vi "Dashboard Main KB.vi"() -> ()   [LabVIEW 2014]
uses:
  Typedefs/StackerStates.ctl
  Typedefs/Arm States.ctl
  Typedefs/ClawStates.ctl
  <vilib>/Rock Robotics/Network Tables/SD Read Boolean.vi
  <vilib>/Rock Robotics/Network Tables/SD Read Number.vi
  <vilib>/Rock Robotics/Network Tables/SD Read String Array.vi
panel:
  out "Claw On":bool
  out "Intake On":bool
  out "Right Throttle":dbl
  out "Comp Bot":bool
  out "Intake Sensor Enabled":bool
  out "Number of Totes":u8
  out "Compressor On":bool
  out "Intake Sees Tote":bool
  out "Stacker Sees Tote":bool
  out "Tusks Up":bool
  out "Stacker On":bool
  out "Compressor Enabled":bool
  out "Stacker State to Index":T1
  out "Arm State":T2
  out "Claw State":T3
  out "Auto Mode":string
  out "Left Throttle":dbl
  out "Claw Sees Can":bool
  in  "TCP":refnum<k5>
  out "Camera IP":string
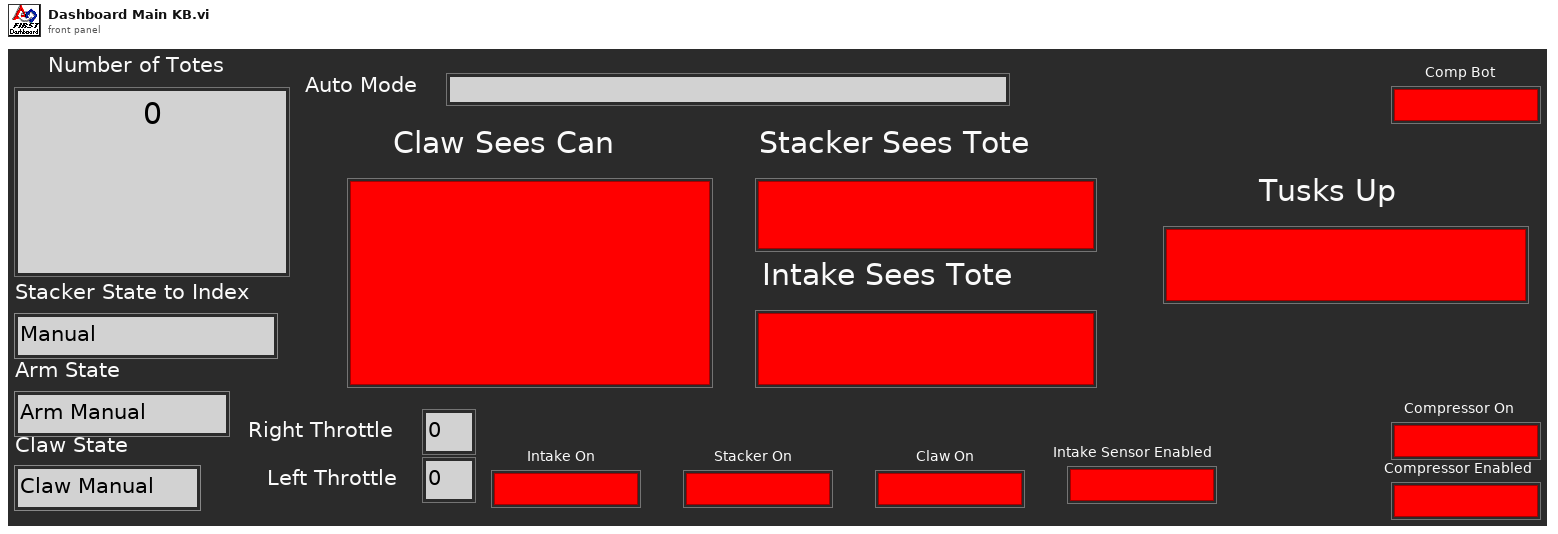
[diagram p1: front panel]
types:
  T1 = typedef "StackerStates.ctl" = enum16{"Manual ", "Hold", "Hold5", "Hold6", "GetTote", "DropStack", "Wait for Up", "DecideHold", "DownTimerPeriod", "Prep Intake for Drop", "Check Arm before 5", "Make Arm ready for 5", "Check Arm before 6", "Make Arm ready for 6", "Delay for 5", "Delay for 6"}
  T2 = typedef "Arm States.ctl" = enum16{"Arm Manual ", "Ground", "Step", "1 Tote", "2 Tote", "3 Tote", "4 Tote", "5 Tote", "6 Tote", "Flip Can", "Grab Can in auto"}
  T3 = typedef "ClawStates.ctl" = enum16{"Claw Manual ", "Claw Open", "Claw Closed", "Claw Slight Open", "Tote Get"}
  T4 = cluster{"Error Strings":string, "Disable Counts":cluster{u16, u16}, "Rail Faults":cluster{u16, u16, u16}, "Robot IP":string, "DB Mode":u8, "Event Info":cluster{"Name":string, "Type":u8, "Number":u16, "Replay":u8}, "Camera Addr":string}
  T5 = cluster{"Storage":cluster{"Disk Free":u64, "RAM Block":u32, "RAM free":u32}, "CPU Utilization":cluster{"CPU % ISR":sgl, "CPU % Time Crit":sgl, "CPU % Timed Str":sgl, "CPU % High":sgl, "CPU % Above":sgl, "CPU % Normal":sgl, "CPU % Low":sgl}, "CAN":cluster{"% Bus Utilization":sgl, "Bus Off Cnt":u32, "TX_FIFO Full Cnt":u32, "Receive Error Cnt":u8, "Transmit Error Cnt":u8}, "HID":cluster{"HID Outputs":u32, "Rumble Low":u16, "Rumble High":u16}[]}
  T6 = cluster{"Status bits":cluster{"Test Mode":bool, "Autonomous":bool, "Enabled":bool, "Code Start":bool, "Brownout":bool, "Reserved 2":bool, "Reserved 3":bool, "E-Stop":bool}, "Code Trace":cluster{"Disabled":bool, "TeleOp":bool, "Auto":bool, "Test":bool}, "Controller Type":enum16{"unknown", "cRIO", "roboRio"}, "Code?":enum16{"unknown", "noCode", "code"}, "Battery V":dbl}
  T7 = cluster{"Control Bits":cluster{"TestMode":bool, "Autonomous":bool, "Enabled":bool, "FMS Present":bool, bool, bool, bool, "E-Stop":bool}, "Team Station ":u8, "Countdown":sgl, "Joystick Values":cluster{"Axes":dbl[], "Buttons":bool[], "POVs":i16[]}[]}
  T8 = enum8{"Tele-Op Disabled", "Tele-Op Enabled", "Auto Disabled", "Auto Enabled", "Test Disabled", "Test Enabled", "Disconnected", "No Code", "E-Stop"}
  T9 = cluster{"Axes":dbl[], "Buttons":bool[], "POVs":i16[]}[]
  T10 = cluster{"Axes":dbl[], "Buttons":bool[], "POVs":i16[]}
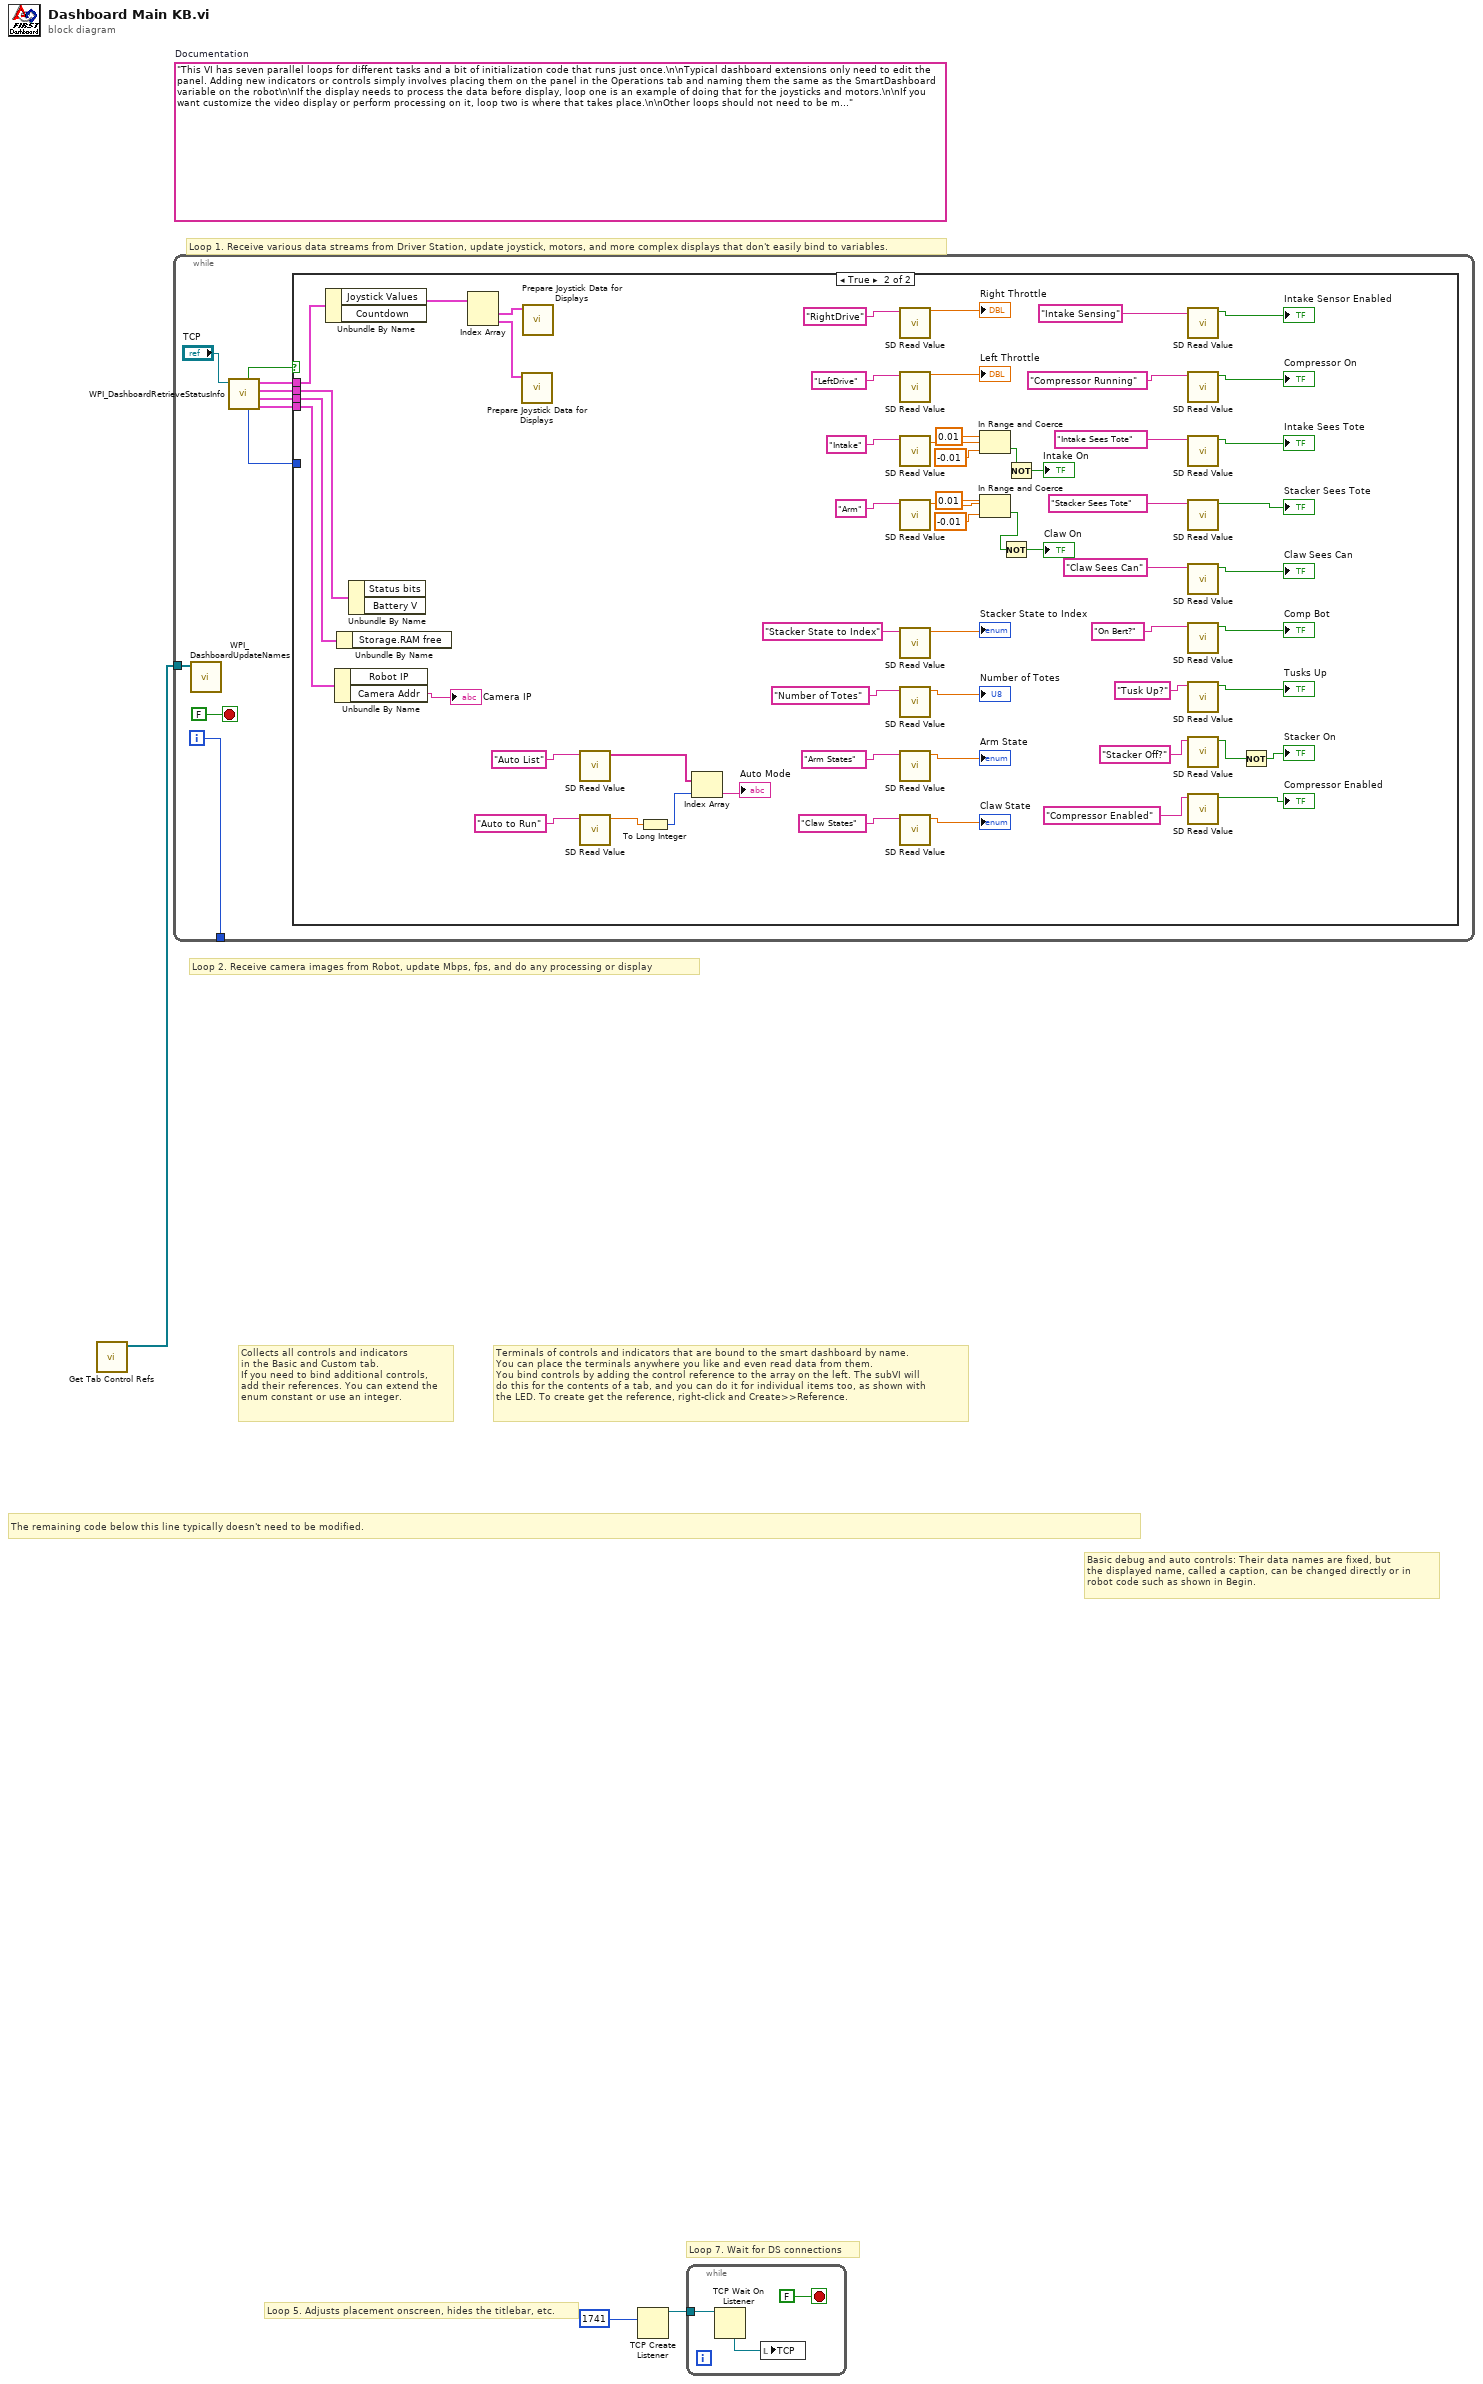
[diagram p0: block diagram]
diagram:
  (unwired) "This VI has seven parallel loops for different tasks and a bit of initialization code that runs just once.\n\nTypical dashboard extensions only need to edit the panel. Adding new indicators or controls simply involves placing them on the panel in the Operations tab and naming them the same as the SmartDashboard variable on the robot\n\nIf the display needs to process the data before display, loop one is an example of doing that for the joysticks and motors.\n\nIf you want customize the video display or perform processing on it, loop two is where that takes place.\n\nOther loops should not need to be modified. They are pretty standard, and document the task they perform."  # Documentation
  # "Loop 7. Wait for DS connections"
  # "Basic debug and auto controls: Their data names are fixed, but\nthe displayed name, called a caption, can be changed directly or in\nrobot code such as shown in Begin."
  # "Collects all controls and indicators\nin the Basic and Custom tab.\nIf you need to bind additional controls,\nadd their references. You can extend the\nenum constant or use an integer."
  # "The remaining code below this line typically doesn't need to be modified."
  # "Terminals of controls and indicators that are bound to the smart dashboard by name.\nYou can place the terminals anywhere you like and even read data from them.\nYou bind controls by adding the control reference to the array on the left. The subVI will\ndo this for the contents of a tab, and you can do it for individual items too, as shown with\nthe LED. To create get the reference, right-click and Create>>Reference."
  # "Loop 5. Adjusts placement onscreen, hides the titlebar, etc."
  # "Loop 1. Receive various data streams from Driver Station, update joystick, motors, and more complex displays that don't easily bind to variables."
  # "Loop 2. Receive camera images from Robot, update Mbps, fps, and do any processing or display"
  n1 = call <vilib>:"Get Tab Control Refs.vi"() -> ("ControlsOnPage"=w3:refnum<vi>[])  [unwired: 11 in]
  n2 = while {
    tunnel: [w12] -> _
    tunnel: w3 -> [w6]
    i -> [w12]
    stop <- FALSE stop-if-true
    n3 = call <vilib>:"WPI_DashboardUpdateNames.vi"("Controls on Tab"=w6) -> ()  [unwired: 11 in]
    n4 = call <vilib>:"WPI_DashboardRetrieveStatusInfo.vi"("TCP Cnx"="TCP") -> ("Power and Errors"=w7:T4, "Robot Metrics"=w10:T5, "Status Info"=w11:T6, "Control Info"=w8:T7, "Robot Mode"=w5:T8, "Process?"=w9:bool)  [unwired: 5 in]
    n5 = case shown="True" w9 {
      tunnel: w11 -> [_ w70]
      tunnel: w10 -> [_ w69]
      tunnel: w8 -> [_ w68]
      tunnel: w7 -> [_ w67]
      tunnel: w5 -> [_ _]
      frame False {
      }
      frame True {
        n6 = Unbundle By Name(w68) -> ("Joystick Values"=w66:T9)  [unwired: 1 out]
        n7 = Unbundle By Name(w67) -> ("Camera Addr"=→"Camera IP":string)  [unwired: 1 out]
        n8 = Unbundle By Name(w69) -> ()  [unwired: 1 out]
        n9 = Unbundle By Name(w70) -> ()  [unwired: 2 out]
        n10 = Index Array(array=w66) -> (element #1=w65:T10, element #2=w63:T10)  [unwired: 2 in]
        n11 = call "Prepare Joystick Data for Displays.vi"("Joystick Values"=w63) -> ()  [unwired: 8 in, 3 out]
        n12 = call "Prepare Joystick Data for Displays.vi"("Joystick Values"=w65) -> ()  [unwired: 8 in, 3 out]
        n13 = call-poly <vilib>:"SD Read Value.vi"("Name"="Auto List") -> ("String Array"=w31:string[])  [unwired: 9 in, 1 out]
        n14 = call-poly <vilib>:"SD Read Value.vi"("Name"="Auto to Run") -> ("Numeric"=w30:dbl)  [unwired: 8 in, 2 out]
        n15 = To Long Integer(number=w30) -> (32bit integer=w29:i32)
        n16 = Index Array(array=w31, index=w29) -> (element=→"Auto Mode":string)
        n17 = call-poly <vilib>:"SD Read Value.vi"("Name"="RightDrive") -> ("Numeric"=→"Right Throttle":dbl)  [unwired: 8 in, 2 out]
        n18 = call-poly <vilib>:"SD Read Value.vi"("Name"="LeftDrive") -> ("Numeric"=→"Left Throttle":dbl)  [unwired: 8 in, 2 out]
        n19 = call-poly <vilib>:"SD Read Value.vi"("Name"="Intake") -> ("Numeric"=w25:dbl)  [unwired: 8 in, 2 out]
        n20 = call-poly <vilib>:"SD Read Value.vi"("Name"="Arm") -> ("Numeric"=w20:dbl)  [unwired: 8 in, 2 out]
        n21 = call-poly <vilib>:"SD Read Value.vi"("Name"="Stacker State to Index") -> ("Numeric"=→"Stacker State to Index":dbl)  [unwired: 8 in, 2 out]
        n22 = call-poly <vilib>:"SD Read Value.vi"("Name"="Number of Totes") -> ("Numeric"=→"Number of Totes":dbl)  [unwired: 8 in, 2 out]
        n23 = call-poly <vilib>:"SD Read Value.vi"("Name"="Arm States") -> ("Numeric"=→"Arm State":dbl)  [unwired: 8 in, 2 out]
        n24 = call-poly <vilib>:"SD Read Value.vi"("Name"="Claw States") -> ("Numeric"=→"Claw State":dbl)  [unwired: 8 in, 2 out]
        n25 = In Range and Coerce(upper limit=0.01, x=w25, lower limit=-0.01 ("upper limit")) -> (In Range?=w18:bool)  [unwired: 1 out]
        n26 = In Range and Coerce(upper limit=0.01, x=w20, lower limit=-0.01 ("upper limit")) -> (In Range?=w16:bool)  [unwired: 1 out]
        n27 = Not(x=w16) -> (.not. x?=→"Claw On":bool)
        n28 = Not(x=w18) -> (.not. x?=→"Intake On":bool)
        n29 = call-poly <vilib>:"SD Read Value.vi"("Name"="Intake Sensing") -> ("Boolean"=→"Intake Sensor Enabled":bool)  [unwired: 8 in, 2 out]
        n30 = call-poly <vilib>:"SD Read Value.vi"("Name"="Compressor Running") -> ("Boolean"=→"Compressor On":bool)  [unwired: 8 in, 2 out]
        n31 = call-poly <vilib>:"SD Read Value.vi"("Name"="Intake Sees Tote") -> ("Boolean"=→"Intake Sees Tote":bool)  [unwired: 8 in, 2 out]
        n32 = call-poly <vilib>:"SD Read Value.vi"("Name"="Stacker Sees Tote") -> ("Boolean"=→"Stacker Sees Tote":bool)  [unwired: 8 in, 2 out]
        n33 = call-poly <vilib>:"SD Read Value.vi"("Name"="Claw Sees Can") -> ("Boolean"=→"Claw Sees Can":bool)  [unwired: 8 in, 2 out]
        n34 = call-poly <vilib>:"SD Read Value.vi"("Name"="On Bert?") -> ("Boolean"=→"Comp Bot":bool)  [unwired: 8 in, 2 out]
        n35 = call-poly <vilib>:"SD Read Value.vi"("Name"="Tusk Up?") -> ("Boolean"=→"Tusks Up":bool)  [unwired: 8 in, 2 out]
        n36 = call-poly <vilib>:"SD Read Value.vi"("Name"="Stacker Off?") -> ("Boolean"=w14:bool)  [unwired: 8 in, 2 out]
        n37 = call-poly <vilib>:"SD Read Value.vi"("Name"="Compressor Enabled") -> ("Boolean"=→"Compressor Enabled":bool)  [unwired: 8 in, 2 out]
        n38 = Not(x=w14) -> (.not. x?=→"Stacker On":bool)
      }
    }
  }
  n39 = TCP Create Listener(10:u16 1741 ("timeout ms (25000)")) -> (3:w1:refnum<k5>)  [unwired: 4 in, 2 out]
  n40 = while {
    tunnel: w1 -> [w72]
    stop <- FALSE stop-if-true
    n41 = TCP Wait On Listener(11:w72) -> (4:w71:refnum<k5>)  [unwired: 3 in, 4 out]
    n42 = local write "TCP"(w71) -> ()
  }
